vi "TimerHelper.vi"(0 "Start":bool, 5 "Pause/Resume":bool, 7 "Reset":bool, 9 "Stop":bool) -> (4 "Clock":dbl format="%#_6f")   [LabVIEW 2016, in "Timer.lvlib"]
doc: "Basic stopwatch"
uses:
  Timer.lvlib
panel:
  # "STOPWATCH"
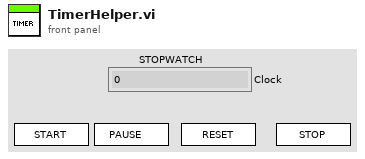
[diagram p1: front panel]
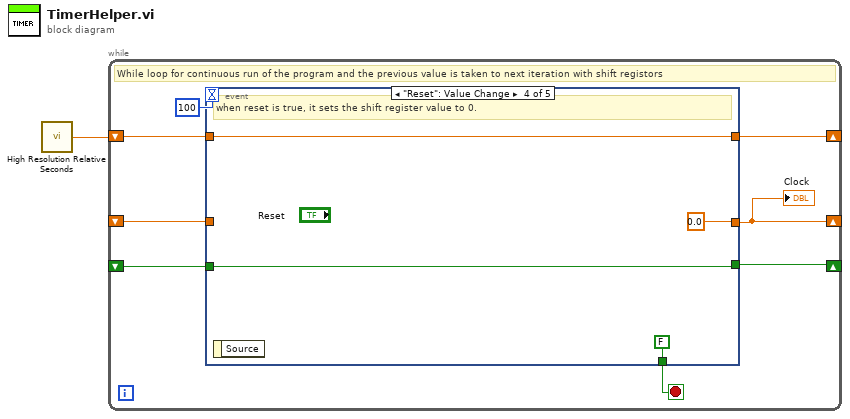
[diagram p0: block diagram]
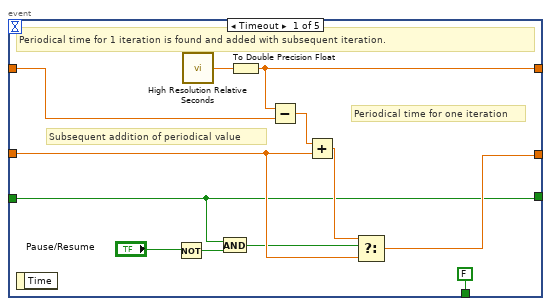
[diagram p2: hidden frame]
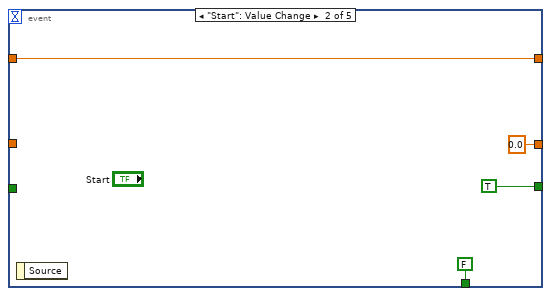
[diagram p3: hidden frame]
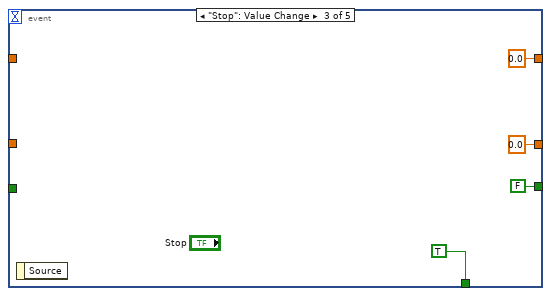
[diagram p4: hidden frame]
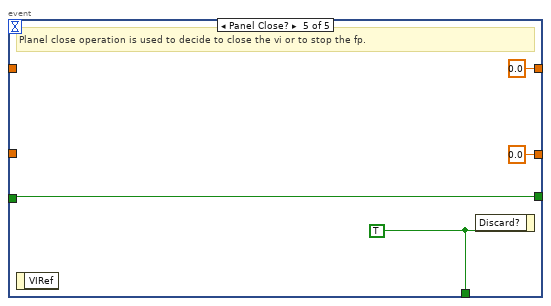
[diagram p5: hidden frame]
diagram:
  n1 = call <vilib>:"High Resolution Relative Seconds.vi"() -> ("relative seconds"=w1:dbl)
  n2 = while {
    shift-right: [w5] -> _
    shift-left: _ -> [w9]
    shift-right: [w8] -> _
    shift-left: w1 -> [w7]
    shift-right: [w3] -> _
    shift-left: _ -> [w2]
    stop <- w4 stop-if-true
    # "While loop for continuous run of the program and the previous value is taken to next iteration with shift registors"
    n3 = event shown="[3] \"Reset\": Value Change" {
      selector: _ -> [_ _ _ _ _]
      dyn-events: _ -> [_ _ _ _ _]
      timeout: 100 -> [_ _ _ _ _]
      tunnel: w9 -> [w21 _ _ _ _]
      tunnel: [w20 w25 0.0 ("relative seconds") w33 0.0 ("relative seconds")] -> w8
      tunnel: [w14 0.0 0.0 0.0 0.0] -> w5
      tunnel: w7 -> [w19 w25 _ w33 _]
      tunnel: w2 -> [w11 _ _ w31 w36]
      tunnel: [FALSE FALSE TRUE FALSE w37] -> w4
      tunnel: [w11 TRUE FALSE w31 w36] -> w3
      event Timeout {
        # "Subsequent addition of periodical value"
        # "Periodical time for one iteration"
        # "Periodical time for 1 iteration is found and added with subsequent iteration."
        n4 = event-data() -> ()  [unwired: 1 in, 1 out]
        n5 = Not(x="Pause/Resume") -> (.not. x?=w13:bool)
        n6 = call <vilib>:"High Resolution Relative Seconds.vi"() -> ("relative seconds"=w18:dbl)
        n7 = And(x=w11, y=w13) -> (x .and. y?=w12:bool)
        n8 = To Double Precision Float(number=w18) -> (double precision float=w20:dbl)
        n9 = Subtract(x=w20, y=w19) -> (x-y=w16:dbl)
        n10 = Add(x=w16, y=w21) -> (x+y=w17:dbl)
        n11 = Select(t=w17, s=w12, f=w21) -> (s? t:f=w14:dbl)
      }
      event "Start": Value Change {
        n12 = event-data() -> ()  [unwired: 1 in, 1 out]
      }
      event "Stop": Value Change {
        n13 = event-data() -> ()  [unwired: 1 in, 1 out]
      }
      event "Reset": Value Change {
        # "when reset is true, it sets the shift register value to 0."
        n14 = event-data() -> ()  [unwired: 1 in, 1 out]
      }
      event Panel Close? {
        w37 = TRUE
        # "Planel close operation is used to decide to close the vi or to stop the fp."
        n15 = event-data() -> ()  [unwired: 1 in, 1 out]
        n16 = event-data("Discard?"=w37) -> ()  [unwired: 1 in, 1 out]
      }
    }
    "Clock" <- w5
  }
